vi "New-Update Assertion.vi"(8 "error in (no error)":errorcluster, 10 "Assertion":refnum<class "TestManagerMsg.Assertion.lvclass">, 11 "Test Event Storage in":refnum<class "Test Event Storage.lvclass">) -> (0 "error out":errorcluster, 2 "Assert ID":string, 3 "Test Event Storage out":refnum<class "Test Event Storage.lvclass">)   [LabVIEW 2020, in "Caraya.lvlib" / "Test Event Storage.lvclass"]
uses:
  Test Event Storage.lvclass
  Test Manager Message Assertion/TestManagerMsg.Assertion.lvclass
  C:/projects/caraya/src/classes/Test Manager Message/TestManagerMsg.lvclass
  Test Event Storage.lvclass/Test Event Storage.ctl
  assert store -- cluster.ctl
  Test Manager Message Verbose/TestManagerMsg.Verbose.lvclass
  Test Manager Message/TestManagerMsg.lvclass/TestManagerMsg.ctl
  Test Manager Message/TestManagerMsg.lvclass
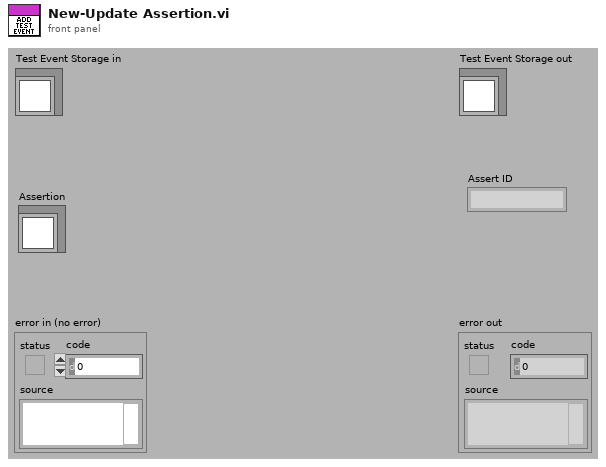
[diagram p1: front panel]
types:
  T1 = typedef "Caraya.lvlib/Test Event Storage.lvclass/assert store -- cluster.ctl" = cluster{"Assertion":refnum<class "TestManagerMsg.Assertion.lvclass">, "Explanation":refnum<class "TestManagerMsg.Verbose.lvclass">, "properties":variant, "measurements":variant, "user-defined":variant}
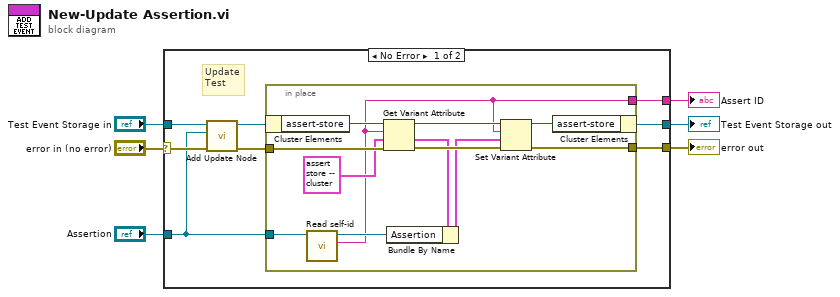
[diagram p0: block diagram]
diagram:
  n1 = case shown="No Error" "error in (no error)" {
    selector: "error in (no error)" -> [w12 w28]
    tunnel: [w14 w28] -> w5
    tunnel: [w13 w27] -> w3
    tunnel: "Test Event Storage in" -> [w10 w27]
    tunnel: [w11 _] -> w2
    tunnel: "Assertion" -> [w9 _]
    frame No Error {
      # "Update\nTest"
      n2 = call "Add Update Node.vi"("error in (no error)"=w12, "Assertion"=w9, "Test Event Storage in"=w10) -> ("error out"=w8:errorcluster, "Test Event Storage out"=w7:refnum<class "Test Event Storage.lvclass">)  [unwired: 6 in, 1 out]
      n3 = in-place {
        in-place-border: w8 -> [w21]
        in-place-border: [w15] -> w14
        in-place-border: [w16] -> w11
        in-place-border: w9 -> [w25]
        n4 = in-place-cluster #1(w7) -> ("assert-store"=w23:variant)
        n5 = call "Read self-id.vi"("TestManagerMsg in"=w25) -> ("self-id"=w16:string, "TestManagerMsg out"=w24:refnum<class "TestManagerMsg.Assertion.lvclass">)  [unwired: 9 in]
        n6 = Get Variant Attribute(Variant=w23, name=w16, default value (empty Variant)=T1 {"Assertion"=refnum, "Explanation"=refnum, "properties"=variant, "measurements"=variant, "user-defined"=variant} ("assert-store"), error in=w21) -> (duplicate Variant=w22:variant, value=w18:T1, error out=w20:errorcluster)  [unwired: 1 out]
        n7 = Bundle By Name(cluster=w18, "Assertion"=w24) -> (w17:T1)
        n8 = Set Variant Attribute(Variant=w22, name=w16, value=w17, error in=w20) -> (Variant out=w26:variant, error out=w15:errorcluster)  [unwired: 1 out]
        n9 = in-place-cluster #1("assert-store"=w26) -> (w13:refnum<class "Test Event Storage.lvclass">)
      }
    }
    frame Error {
    }
  }
  "error out" <- w5
  "Test Event Storage out" <- w3
  "Assert ID" <- w2
